vi "AB_Set_Destination_CORE.vi"(8 "error in (no error)":errorcluster, 10 "destination index":i32, 11 "Source in":refnum<class "AB_Source.lvclass">) -> (0 "error out":errorcluster, 3 "Source out":refnum<class "AB_Source.lvclass">)   [LabVIEW 2020]
uses:
  <vilib>/AppBuilder/AB_Classes/Source/AB_Source.lvclass
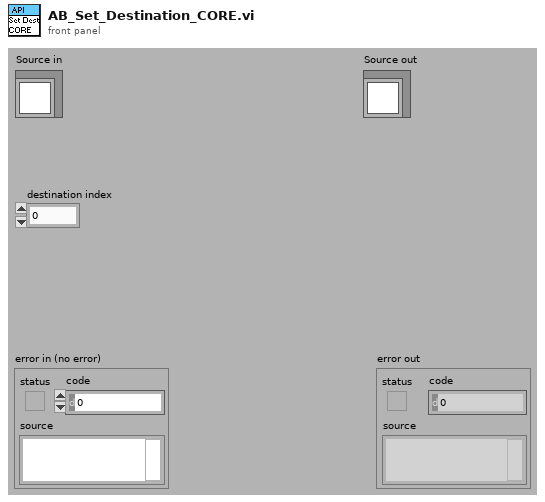
[diagram p1: front panel]
types:
  T1 = typedef "AB_Source.ctl" = cluster{"path":path, "itemID":string, "parentIndex":i32, "sourceInclusion":T2, "destinationIndex":i32, "properties":T3[], "newName":string, "lvfile":bool, "valid":bool, "eng_inBuild":bool, "eng_isNonVILink":bool, "Amalgamation":bool, "Amalgamation Piece":bool, "eng_delimitedName":string, "preventRename":bool}
  T2 = typedef "AB_Source_Inclusion.ctl" = enum16{"IncludeIfReferenced", "Include", "Exclude", "TopLevel"}
  T3 = typedef "AB_Source_Properties.ctl" = cluster{"sourcePropertyType":T4, "value":variant}
  T4 = typedef "AB_Source_Property_Type.ctl" = enum16{"Remove block diagram", "Remove front panel", "Password", "Window has title bar", "Show menu bar", "Show vertical scroll bar", "Show horizontal scroll bar", "Show toolbar", "Show Abort button", "Show fp when called", "Window behavior", "Allow user to close window", "Window run-time position", "Run when opened", "Allow debugging", "Auto error handling", "Generate guard code", "Use stack variables", "Expression folding", "Integer only", "Inline subVI"}
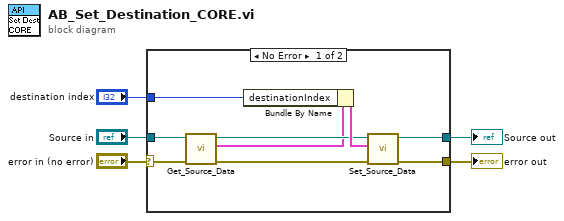
[diagram p0: block diagram]
diagram:
  n1 = case shown="No Error" "error in (no error)" {
    selector: "error in (no error)" -> [w10 w16]
    tunnel: [w8 w16] -> w4
    tunnel: "destination index" -> [w11 _]
    tunnel: "Source in" -> [w7 w15]
    tunnel: [w6 w15] -> w1
    frame No Error {
      n2 = call <vilib>:"Get_Source_Data.vi"("error in (no error)"=w10, "Class in"=w7) -> ("error out"=w9:errorcluster, "data"=w12:T1, "Class out"=w13:refnum<class "AB_Source.lvclass">)  [unwired: 7 out]
      n3 = Bundle By Name(cluster=w12, "destinationIndex"=w11) -> (w14:T1)
      n4 = call <vilib>:"Set_Source_Data.vi"("error in (no error)"=w9, "data"=w14, "Class in"=w13) -> ("error out"=w8:errorcluster, "Class out"=w6:refnum<class "AB_Source.lvclass">)  [unwired: 7 out]
    }
    frame Error {
    }
  }
  "error out" <- w4
  "Source out" <- w1
